vi "read Sim_iXon Class.vi"(8 "error in (no error)":errorcluster, 11 "SPARC4_Channel in":refnum<class "SPARC4_Channel.lvclass">) -> (0 "error out":errorcluster, 2 "Sim_Ixon_Ultra.lvclass":refnum<class "Sim_Ixon_Ultra.lvclass">, 3 "SPARC4_Channel out":refnum<class "SPARC4_Channel.lvclass">)   [LabVIEW 2018, in "SPARC4_Channel.lvclass"]
uses:
  SPARC4_Channel.lvclass
  Sim_Ixon_Ultra/Sim_Ixon_Ultra.lvclass
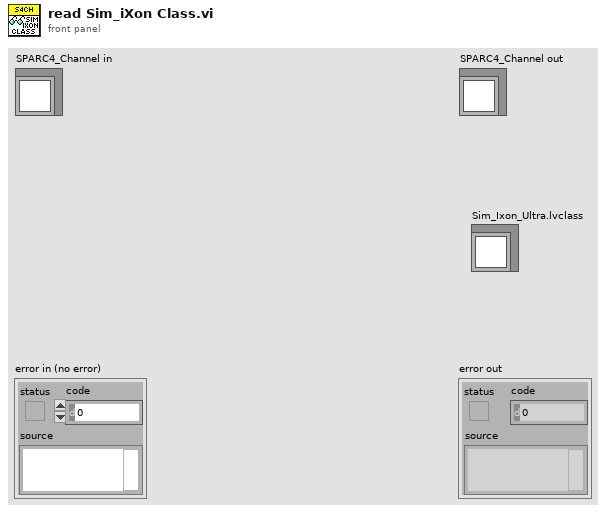
[diagram p1: front panel]
types:
  T1 = cluster{"State Machine.lvclass":refnum<class "State Machine.lvclass">, "RxTx.lvclass":refnum<class "RxTx.lvclass">, "Save_Header_RxTx.lvclass":refnum<class "RxTx.lvclass">, "Status SM.lvclass":refnum<class "State Machine.lvclass">, "Status RxTx.lvclass":refnum<class "RxTx.lvclass">, "servers array":refnum<class "Server.lvclass">[], "Events log file.lvclass":refnum<class "Log File.lvclass">, "Errors log file.lvclass":refnum<class "Log File.lvclass">, "Keywords log file.lvclass":refnum<class "Log File.lvclass">, "Sim_CCD.lvclass":refnum<class "Sim_CCD.lvclass">}
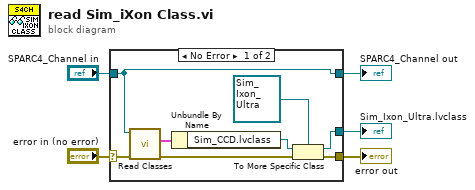
[diagram p0: block diagram]
diagram:
  n1 = case shown="No Error" "error in (no error)" {
    selector: "error in (no error)" -> [w13 w15]
    tunnel: [w6 w15] -> w4
    tunnel: [w12 w14] -> w2
    tunnel: "SPARC4_Channel in" -> [w12 w14]
    tunnel: [w8 _] -> w1
    frame No Error {
      n2 = call-dynamic "Read Classes.vi"("error in (no error)"=w13, "Channel in"=w12) -> ("error out"=w7:errorcluster, "Classes"=w11:T1)  [unwired: 7 in, 1 out]
      n3 = Unbundle By Name(w11) -> ("Sim_CCD.lvclass"=w9:refnum<class "Sim_CCD.lvclass">)
      n4 = To More Specific Class(target class=refnum<class "Sim_Ixon_Ultra.lvclass"> refnum ("Sim_Ixon_Ultra.lvclass 2"), reference=w9, error in=w7) -> (specific class reference=w8:refnum<class "Sim_Ixon_Ultra.lvclass">, error out=w6:errorcluster)
    }
    frame Error {
    }
  }
  "error out" <- w4
  "SPARC4_Channel out" <- w2
  "Sim_Ixon_Ultra.lvclass" <- w1
